vi "Create Directory Recursive.vi"(4 "error in":errorcluster, 7 "directory":path) -> (0 "error out":errorcluster, 3 "directory copy":path)   [LabVIEW 2015, in "Car Wash.lvlib" / "Tools_String.lvlib"]
uses:
  Tools_String.lvlib
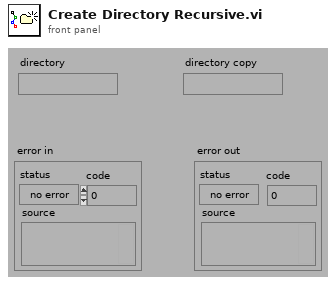
[diagram p1: front panel]
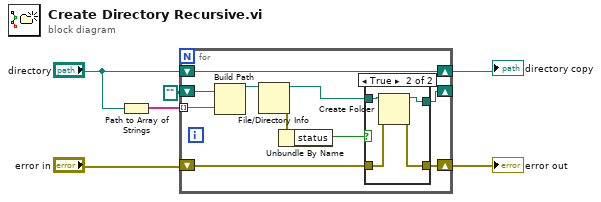
[diagram p0: block diagram]
diagram:
  n1 = Path to Array of Strings(0:"directory") -> (2:w2:string[])  [unwired: 1 out]
  n2 = for {
    shift-right: [w12] -> _
    shift-left: path "" -> [w16]
    tunnel: w2 -> [w15] mode=indexing
    shift-right: [w10] -> w5
    shift-left: "directory" -> [w10]
    shift-right: [w8] -> w3
    shift-left: "error in" -> [w9]
    n3 = Build Path(base path=w16, name or relative path=w15) -> (appended path=w14:path)
    n4 = File/Directory Info(path=w14) -> (path out=w13:path, error out=w11:errorcluster)  [unwired: 1 in, 5 out]
    n5 = Unbundle By Name(w11) -> ("status"=w7:bool)
    n6 = case shown="True" w7 {
      tunnel: [w18 w22] -> w12
      tunnel: w13 -> [w18 w21]
      tunnel: w9 -> [w17 w20]
      tunnel: [w17 w19] -> w8
      frame False {
      }
      frame True {
        n7 = Create Folder(path (use dialog)=w21, error in=w20) -> (created path=w22:path, error out=w19:errorcluster)  [unwired: 2 out]
      }
    }
  }
  "directory copy" <- w5
  "error out" <- w3
